vi "Polynomial_kernel.vi"(8 "error in":errorcluster caption="entrée d'erreur", 9 "Y":string[][](array[string]), 10 "X":string[][](array[string]), 11 "polynomial_kernel":T2={"degree"=3, "gamma"="None", "coef0"=1.0}) -> (0 "error out":errorcluster caption="sortie d'erreur", 3 "Data":T1)   [LabVIEW 2020]
doc: "Compute the polynomial kernel between X and Y :\n\nK(X, Y) = (gamma <X, Y> + coef0)^degree\n\n\nParameters : \n\n- X : ndarray of shape (n_samples_1, n_features)\n\n- Y : ndarray of shape (n_samples_2, n_features)\n\n- degree : int, default 3\n\n- gamma : float, default None\nif None, defaults to 1.0 / n_features\n\n- coef0 : float, default 1\n\nReturns : \n\n- Gram matrix : array of shape (n_samples_1, n_samples_2)"
uses:
  Polynomial_kernel.lvclass
panel:
  out "Polynomial_kernel.lvclass":refnum<class "Polynomial_kernel.lvclass">
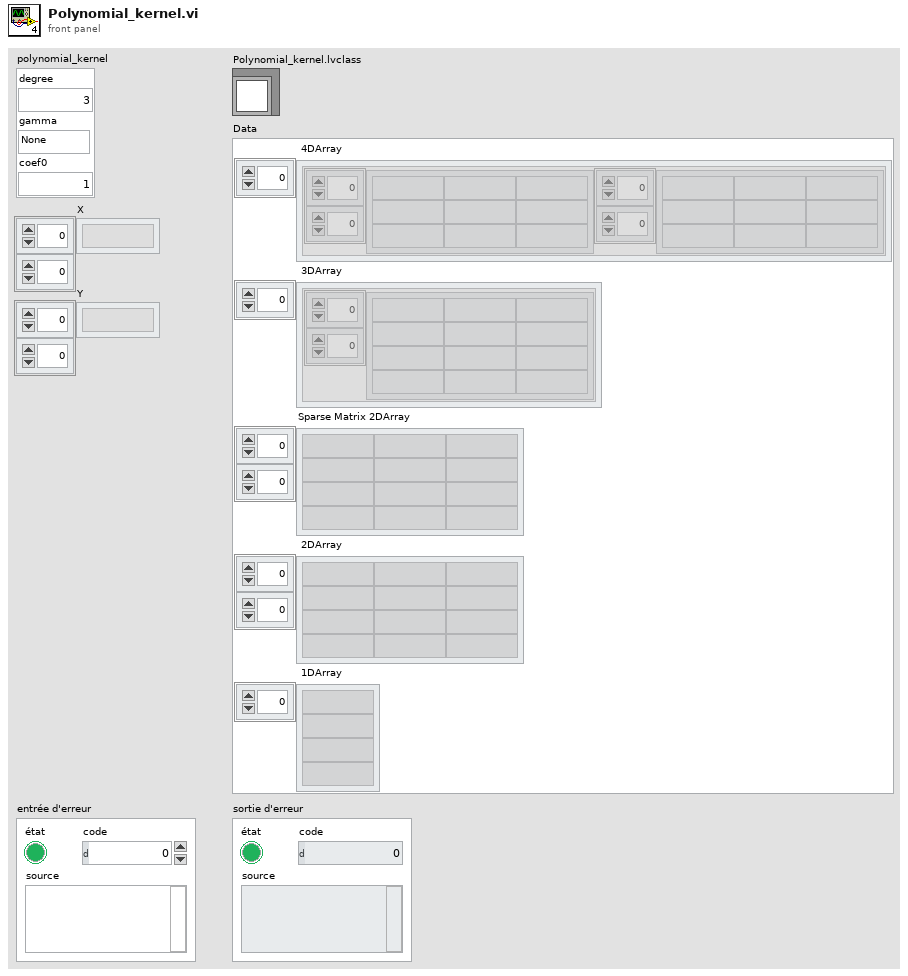
[diagram p1: front panel]
types:
  T1 = cluster{" 4DArray":cluster{"1":string[][], "2":string[][]}[], " 3DArray":cluster{"Tableau":string[][]}[], "Sparse Matrix 2DArray":string[][], " 2DArray":string[][], " 1DArray":string[]}
  T2 = cluster{"degree":i32, "gamma":string, "coef0":dbl}
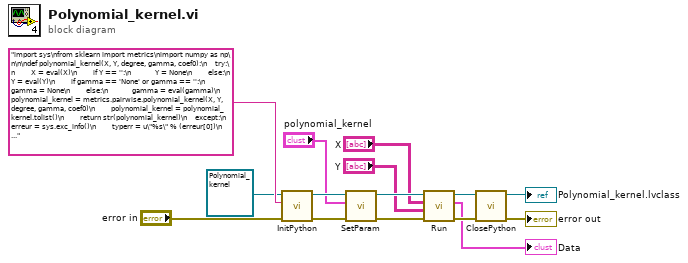
[diagram p0: block diagram]
diagram:
  n1 = call-dynamic "InitPython.vi"("error in (no error)"="error in", "Python Instruction"="import sys\nfrom sklearn import metrics\nimport numpy as np\n\n\ndef polynomial_kernel(X, Y, degree, gamma, coef0):\n    try:\n        X = eval(X)\n        if Y == '':\n            Y = None\n        else:\n            Y = eval(Y)\n        if gamma == 'None' or gamma == '':\n            gamma = None\n        else:\n            gamma = eval(gamma)\n        polynomial_kernel = metrics.pairwise.polynomial_kernel(X, Y, degree, gamma, coef0)\n        polynomial_kernel = polynomial_kernel.tolist()\n        return str(polynomial_kernel)\n    except:\n        erreur = sys.exc_info()\n        typerr = u\"%s\" % (erreur[0])\n        typerr = typerr[typerr.find(\"'\")+1:typerr.rfind(\"'\")]\n        msgerr = u\"%s\" % (erreur[1])\n        message = str('/!\\\\ {0} : {1}'. format(typerr,msgerr))\n        return message", "Scikit-learn en entrée"=refnum<class "Polynomial_kernel.lvclass"> refnum ("Polynomial_kernel.lvclass")) -> ("error out"=w11:errorcluster, "Scikit-learn en sortie"=w13:refnum<class "Polynomial_kernel.lvclass">)  [unwired: 7 in]
  n2 = call-dynamic "SetParam.vi"("error in (no error)"=w11, "polynomial_kernel"="polynomial_kernel", "Polynomial_kernel.lvclass"=w13) -> ("error out"=w8:errorcluster, "Polynomial_kernel.lvclass"=w9:refnum<class "Polynomial_kernel.lvclass">)  [unwired: 7 in]
  n3 = call-dynamic "Run.vi"("error in (no error)"=w8, "Y"="Y", "X"="X", "Polynomial_kernel.lvclass"=w9) -> ("error out"=w7:errorcluster, "Data"=→"Data":T1, "Polynomial_kernel.lvclass"=w6:refnum<class "Polynomial_kernel.lvclass">)  [unwired: 5 in]
  n4 = call-dynamic "ClosePython.vi"("error in (no error)"=w7, "Scikit-learn en entrée"=w6) -> ("error out"=→"error out":errorcluster, "Scikit-learn en sortie"=→"Polynomial_kernel.lvclass":refnum<class "Polynomial_kernel.lvclass">)  [unwired: 8 in]
